vi "Sub-VI_Erros-Soma-Furo.vi"(0 "Furo no Tanque 6":bool, 1 "Boolean 3":bool, 2 "Boolean 4":bool, 5 "Anterior":bool, 7 "Furo no Tanque 5":bool, 9 "Furo no Tanque":bool, 12 "Furo no Tanque 4":bool, 13 "Furo no Tanque 3":bool, 14 "Furo no Tanque 2":bool) -> (4 "Boolean out":bool)   [LabVIEW 2019]
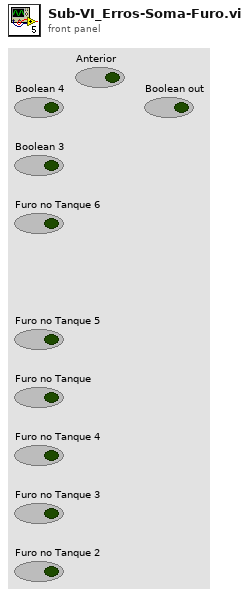
[diagram p1: front panel]
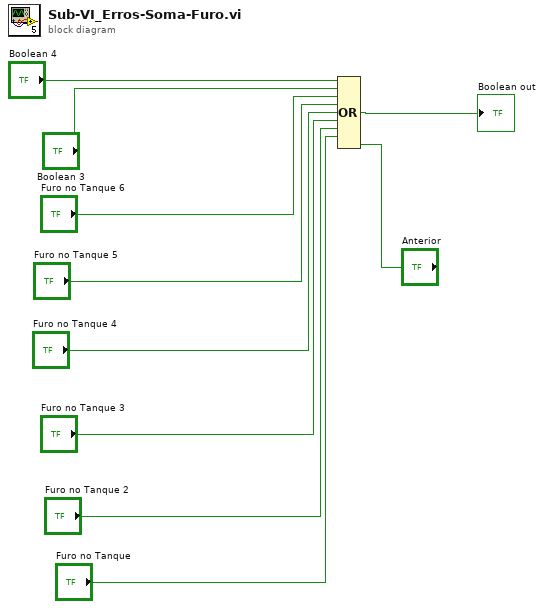
[diagram p0: block diagram]
diagram:
  n1 = Compound Arithmetic op=OR("Boolean 4", "Boolean 3", "Furo no Tanque 6", "Furo no Tanque 5", "Furo no Tanque 4", "Furo no Tanque 3", "Furo no Tanque 2", "Furo no Tanque", "Anterior") -> (→"Boolean out":bool)
